vi "comet_thermo_get_value.vi"(8 "error in":errorcluster, 10 "timeout (5000)":i32=5000, 11 "thermo in":T1={"type"=enum."COMET Tx5xx (ethernet)", "comment"="", "tag"="", "refresh"=0.0, "IP"="", "port"=0, "VISA"="", "last readout"=timestamp(0 s since 1904-01-01), "TCP ref"=refnum, "VISA sess"="", "idn"="", "press"=0.0, "RH"=0.0, "temp"=0.0, "pres cor"=[], "RH cor"=[], "temp cor"=[], "try left"=0, "failed"=FALSE, "RTD set"=[], "RTD inv"=[], "range"=0.0, "net mode"=enum."MODBUS", "try fail"=enum."Stop trying - return NaN", "timeout [s]"=0.0, "max retries"=0, "sim t [deg]"=0.0, "status"=0} {"status" items=["ok", "retry", "failed"]; "RTD inv" format="%.1f"; "RTD set" format="%.1f"; "temp cor" format="%.1f"; "RH cor" format="%.1f"; "pres cor" format="%.1f"; "refresh" min=0.1 max=1000.0 format="%.2f"}) -> (0 "error out":errorcluster, 1 "RH [%]":dbl, 2 "t [C]":dbl, 3 "thermo out":T1={"type"=enum."COMET Tx5xx (ethernet)", "comment"="", "tag"="", "refresh"=5.0, "IP"="", "port"=502, "VISA"="", "last readout"=timestamp(0 s since 1904-01-01), "TCP ref"=refnum, "VISA sess"="", "idn"="", "press"=0.0, "RH"=0.0, "temp"=0.0, "pres cor"=[], "RH cor"=[], "temp cor"=[], "try left"=0, "failed"=FALSE, "RTD set"=[], "RTD inv"=[], "range"=0.0, "net mode"=enum."MODBUS", "try fail"=enum."Stop trying - return NaN", "timeout [s]"=0.0, "max retries"=0, "sim t [deg]"=0.0, "status"=0} {"status" items=["ok", "retry", "failed"]; "RTD inv" format="%.1f"; "RTD set" format="%.1f"; "temp cor" format="%.1f"; "RH cor" format="%.1f"; "pres cor" format="%.1f"; "refresh" min=0.1 max=1000.0 format="%.2f"}, 4 "p [hPa]":dbl, 5 "p4":dbl)   [LabVIEW 2020]
uses:
  thermo.ctl
  thermo_types.ctl
  Thermometer Fail Action.ctl
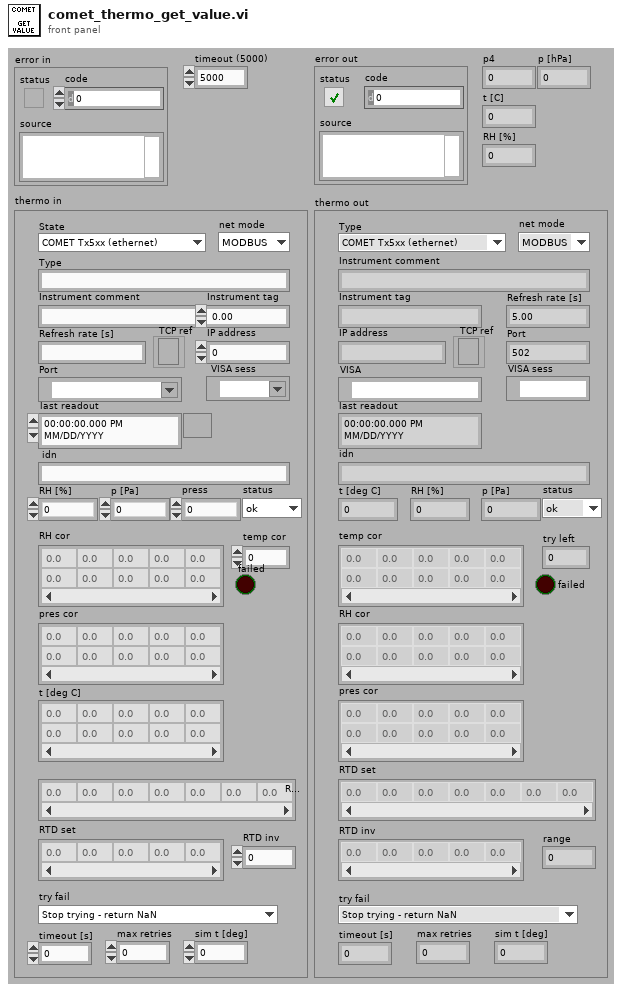
[diagram p1: front panel]
types:
  T1 = typedef "thermo.ctl" = cluster{"type":T2, "comment":string, "tag":string, "refresh":dbl, "IP":string, "port":u16, "VISA":refnum<visa-resource-name>, "last readout":timestamp, "TCP ref":refnum<k5>, "VISA sess":refnum<visa-resource-name>, "idn":string, "press":dbl, "RH":dbl, "temp":dbl, "pres cor":dbl[][], "RH cor":dbl[][], "temp cor":dbl[][], "try left":i32, "failed":bool, "RTD set":dbl[], "RTD inv":dbl[], "range":dbl, "net mode":enum16{"MODBUS", "HTTP"}, "try fail":T3, "timeout [s]":dbl, "max retries":i32, "sim t [deg]":dbl, "status":u16}
  T2 = typedef "thermo_types.ctl" = enum16{"Disabled", "Simulated", "COMET Tx5xx (ethernet)", "Keithley 2002 (GPIB) + RTD", "Agilent 344xx (GPIB) + RTD"}
  T3 = typedef "Thermometer Fail Action.ctl" = enum16{"Stop trying - keep last value", "Stop trying - return NaN", "Generate error - stop sweep"}
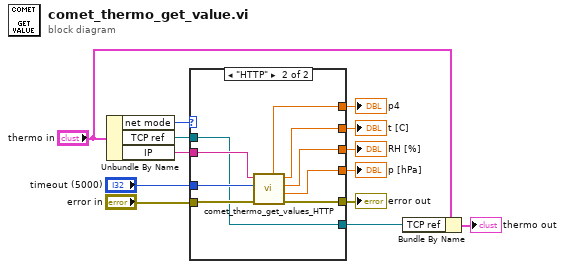
[diagram p0: block diagram]
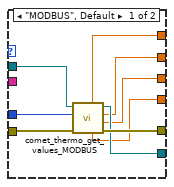
[diagram p2: hidden frame]
diagram:
  n1 = Unbundle By Name("thermo in") -> ("net mode"=w13:enum16{"MODBUS", "HTTP"}, "TCP ref"=w12:refnum<k5>, "IP"=w11:string)
  n2 = case shown="\"HTTP\"" w13 {
    tunnel: "error in" -> [w22 w30]
    tunnel: [w21 w31] -> w9
    tunnel: w12 -> [w20 w23]
    tunnel: "timeout (5000)" -> [w19 w29]
    tunnel: w11 -> [_ w28]
    tunnel: [w16 w27] -> w4
    tunnel: [w15 w26] -> w3
    tunnel: [w14 w25] -> w2
    tunnel: [w18 w24] -> w5
    tunnel: [w17 w23] -> w6
    frame "MODBUS", Default {
      n3 = call "comet_thermo_get_values_MODBUS.vi"("error in"=w22, "Timeout"=w19, "TCP ref in"=w20) -> ("error out"=w21:errorcluster, "RH [%]"=w15:dbl, "t [deg C]"=w16:dbl, "TCP ref out"=w17:refnum<k5>, "p [Pa]"=w14:dbl, "p4"=w18:dbl)  [unwired: 3 in]
    }
    frame "HTTP" {
      n4 = call "comet_thermo_get_values_HTTP.vi"("error in"=w30, "timeout (5000)"=w29, "IP"=w28) -> ("error out"=w31:errorcluster, "p [hPa]"=w25:dbl, "RH [%]"=w26:dbl, "t [C]"=w27:dbl, "p4"=w24:dbl)  [unwired: 4 in]
    }
  }
  "error out" <- w9
  "p4" <- w5
  "t [C]" <- w4
  "RH [%]" <- w3
  "p [hPa]" <- w2
  n5 = Bundle By Name(cluster="thermo in", "TCP ref"=w6) -> (→"thermo out":T1)
